vi "S8300E_SetRTCTime_FromPC.vi"() -> ()   [LabVIEW 2011]
panel:
  out "UUT Msg":string
  out "SFCS Msg":string
  out "VISA resource name out":refnum<visa-resource-name>
  out "begin time":u32
  out "toS8300E_RTC_Data":string
  out "PC_Local_Time":string
  out "PC_DATE_STRING":string
  # "設定標準時間\nSetRTC Time from PC  To S8300E"
  # "2015-6-12"
  # "Error Code:RTC\nError Code:UART"
  # "COM9"
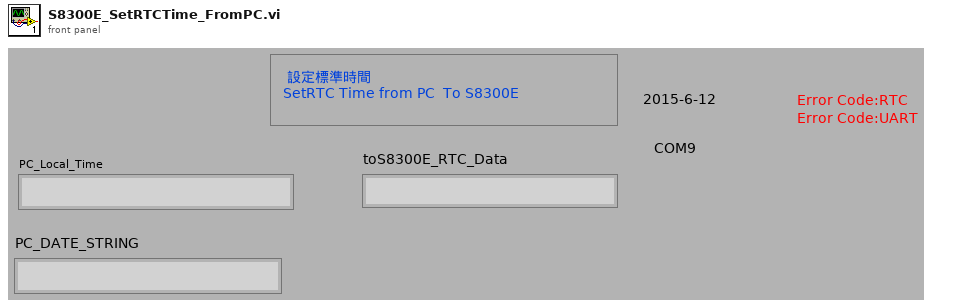
[diagram p1: front panel]
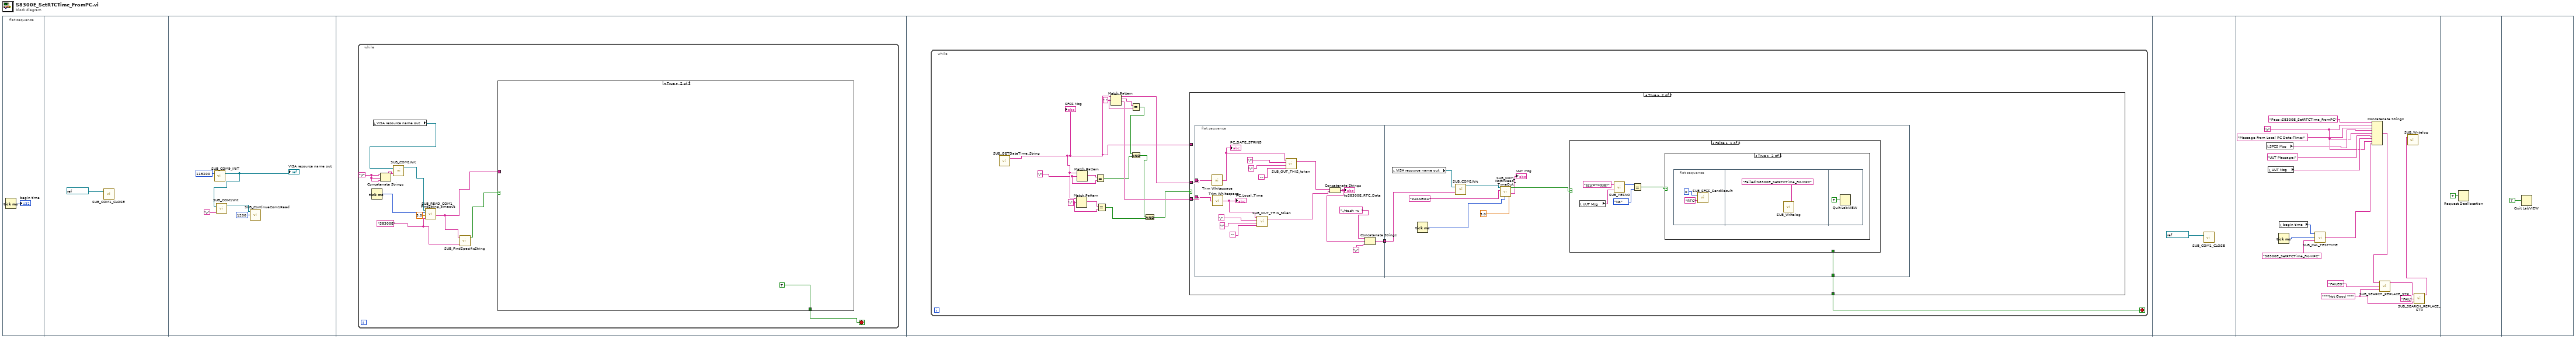
[diagram p0: block diagram]
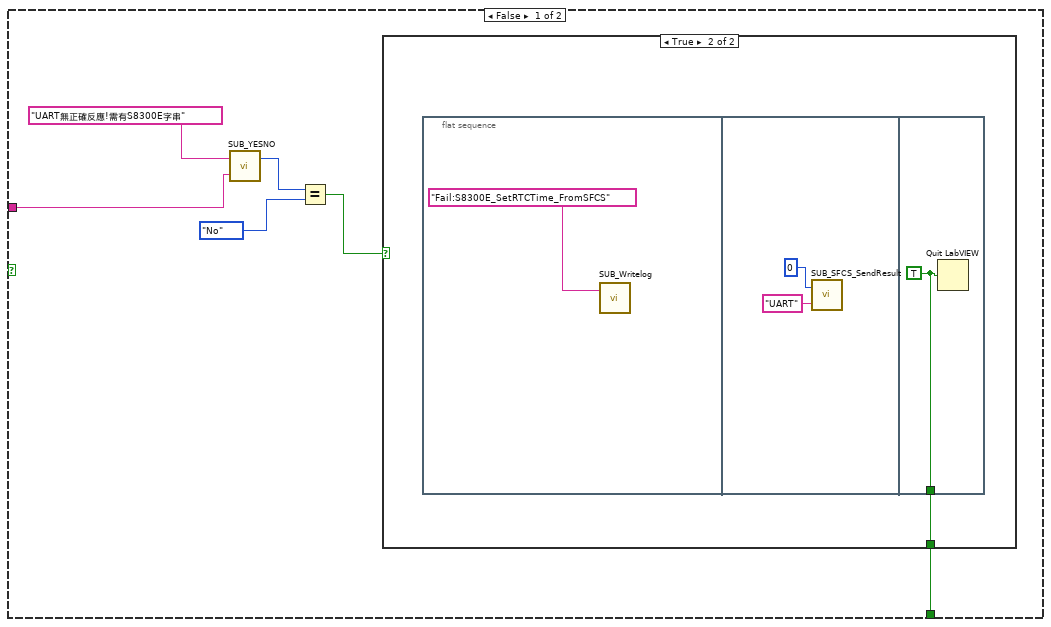
[diagram p2: hidden frame]
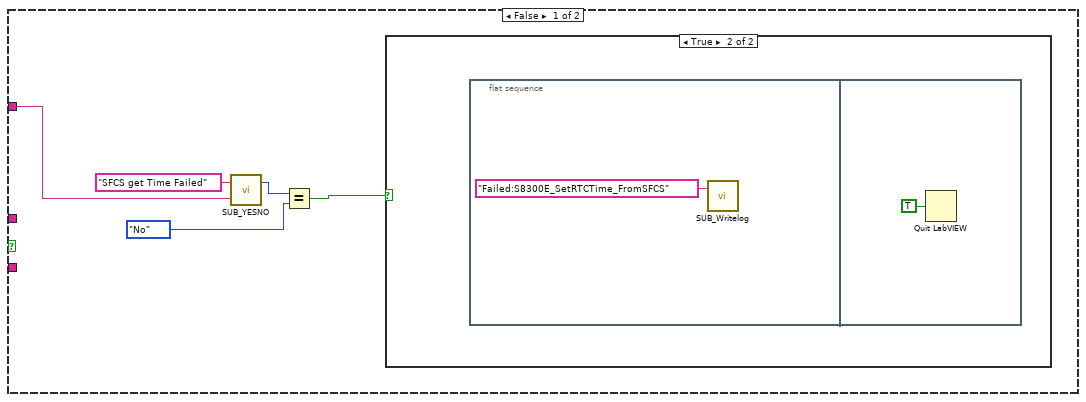
[diagram p4: hidden frame]
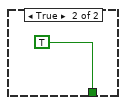
[diagram p7: hidden frame]
diagram:
  n1 = flat-sequence {
    frame #0 {
      n2 = Tick Count (ms)() -> (millisecond timer value=→"begin time":u32)
    }
    frame #1 {
      n3 = call "SUB_COM1_CLOSE.vi"("VISA resource name"=refnum<visa-resource-name> "COM9") -> ()  [unwired: 3 in]
    }
    frame #2 {
      n4 = call "SUB_COM9_INIT.vi"("baud rate"=u32 115200) -> ("VISA resource name out"=w6:refnum<visa-resource-name>)  [unwired: 1 in, 1 out]
      "VISA resource name out" <- w6
      n5 = call "SUB_COM1Wrt.vi"("VISA resource name"=w6, "write buffer"="\r") -> ("duplicate VISA resource name"=w3:refnum<visa-resource-name>)  [unwired: 1 in, 1 out]
      n6 = call "SUB_ContinueCom1Read.vi"("Numeric"=1200, "duplicate VISA resource name 2"=w3) -> ()  [unwired: 1 in, 3 out]
    }
    frame #3 {
      n7 = while {
        stop <- w17 stop-if-true
        w10 = "S8300E" ("Find this String")
        w11 = "\r"
        n8 = Tick Count (ms)() -> (millisecond timer value=w14:u32)
        n9 = local read "VISA resource name out"() -> (w16:refnum<visa-resource-name>)
        n10 = Concatenate Strings(w11, w11, w11) -> (w12:string)
        n11 = call "SUB_COM1Wrt.vi"("VISA resource name"=w16, "write buffer"=w12) -> ("duplicate VISA resource name"=w15:refnum<visa-resource-name>)  [unwired: 1 in, 1 out]
        n12 = call "SUB_READ_COM1_FindString_timeout.vi"("Find this String"=w10, "Timeout Seccond"=3.0, "Begin time"=w14, "duplicate VISA resource name 2"=w15) -> ("Output String"=w9:string)  [unwired: 1 in, 2 out]
        n13 = call "SUB_FindSpecificString.vi"("Find this String"=w10, "String data"=w9) -> ("Found"=w8:bool)  [unwired: 2 in, 1 out]
        n14 = case shown="True" w8 {
          tunnel: w9 -> [w22 _]
          tunnel: [w18 TRUE] -> w17
          frame False {
            n15 = call "SUB_YESNO.vi"("Debug View"=w22, "Status"="UART無正確反應!需有S8300E字串") -> ("yes/no"=w21:enum32{"No Selection", "Yes", "No", "None"})  [unwired: 1 in]
            n16 = Equal?(x=w21, y=enum32{"No Selection", "Yes", "No", "None"}."No") -> (x = y?=w19:bool)
            n17 = case shown="True" w19 {
              tunnel: [_ w24] -> w18
              frame False {
              }
              frame True {
                n18 = flat-sequence {
                  tunnel: [w28] -> w24
                  frame #0 {
                    n19 = call "SUB_Writelog.vi"("Pass/Fail"="Fail:S8300E_SetRTCTime_FromSFCS") -> ()  [unwired: 2 in]
                  }
                  frame #1 {
                    n20 = call "SUB_SFCS_SendResult.vi"("ErrorCode"="UART", "PASS_Fail (1/0)"=i8 0) -> ()  [unwired: 1 out]
                  }
                  frame #2 {
                    w28 = TRUE ("quit? (T)")
                    n21 = Quit LabVIEW(quit? (T)=w28) -> ()
                  }
                }
              }
            }
          }
          frame True {
          }
        }
      }
    }
    frame #4 {
      n22 = while {
        stop <- w33 stop-if-true
        w30 = "/" ("regular expression")
        w38 = ":" ("regular expression")
        w41 = " " ("regular expression")
        n23 = call "SUB_GETDateTime_String.vi"() -> ("date/time string"=w32:string)  [unwired: 3 in]
        "SFCS Msg" <- w32
        n24 = Match Pattern(string=w32, regular expression=w38) -> (match substring=w39:string)  [unwired: 1 in, 3 out]
        n25 = Match Pattern(string=w32, regular expression=w30) -> (match substring=w40:string)  [unwired: 1 in, 3 out]
        n26 = Equal?(x=w40, y=w30) -> (x = y?=w36:bool)
        n27 = Equal?(x=w39, y=w38) -> (x = y?=w31:bool)
        n28 = Match Pattern(string=w32, regular expression=w41) -> (before substring=w44:string, match substring=w42:string, after substring=w43:string)  [unwired: 1 in, 1 out]
        n29 = Equal?(x=w42, y=w41) -> (x = y?=w37:bool)
        n30 = And(x=w37, y=w36) -> (x .and. y?=w35:bool)
        n31 = And(x=w35, y=w31) -> (x .and. y?=w34:bool)
        n32 = case shown="True" w34 {
          tunnel: w44 -> [_ w55]
          tunnel: w43 -> [_ w54]
          tunnel: w32 -> [w45 _]
          tunnel: [_ w53] -> w33
          frame False {
            n33 = call "SUB_YESNO.vi"("Debug View"=w45, "Status"="SFCS get Time Failed") -> ("yes/no"=w48:enum32{"No Selection", "Yes", "No", "None"})  [unwired: 1 in]
            n34 = Equal?(x=w48, y=enum32{"No Selection", "Yes", "No", "None"}."No") -> (x = y?=w46:bool)
            n35 = case shown="True" w46 {
              frame False {
              }
              frame True {
                n36 = flat-sequence {
                  frame #0 {
                    n37 = call "SUB_Writelog.vi"("Pass/Fail"="Failed:S8300E_SetRTCTime_FromSFCS") -> ()  [unwired: 2 in]
                  }
                  frame #1 {
                    n38 = Quit LabVIEW(quit? (T)=TRUE) -> ()
                  }
                }
              }
            }
          }
          frame True {
            n39 = flat-sequence {
              tunnel: w55 -> [w71]
              tunnel: w54 -> [w70]
              tunnel: [w56] -> w52
              tunnel: [w80] -> w53
              tunnel: w52 -> [w78]
              frame #0 {
                n40 = call <vilib>:"Trim Whitespace.vi"("string"=w71) -> ("trimmed string"=w62:string)  [unwired: 1 in]
                "PC_DATE_STRING" <- w62
                n41 = call <vilib>:"Trim Whitespace.vi"("string"=w70) -> ("trimmed string"=w69:string)  [unwired: 1 in]
                "PC_Local_Time" <- w69
                n42 = call "SUB_OUT_THIS_token.vi"("Remove token symbl1 3"="", "Remove token symbl1 2"=":" ("Remove token symbl1"), "Remove token symbl1"="/", "input string"=w69) -> ("result string"=w60:string)  [unwired: 1 in]
                n43 = call "SUB_OUT_THIS_token.vi"("Remove token symbl1 3"="", "Remove token symbl1 2"=":" ("Remove token symbl1"), "Remove token symbl1"="/", "input string"=w62) -> ("result string"=w61:string)  [unwired: 1 in]
                n44 = Concatenate Strings(w61, w60) -> (w57:string)
                "toS8300E_RTC_Data" <- w57
                n45 = Concatenate Strings("./rtc.sh -w  ", w57, "\r") -> (w56:string)
              }
              frame #1 {
                n46 = local read "VISA resource name out"() -> (w79:refnum<visa-resource-name>)
                n47 = Tick Count (ms)() -> (millisecond timer value=w74:u32)
                n48 = call "SUB_COM1Wrt.vi"("VISA resource name"=w79, "write buffer"=w78) -> ("duplicate VISA resource name"=w77:refnum<visa-resource-name>)  [unwired: 1 in, 1 out]
                n49 = call "SUB_COM_NoErrRead_TimeOut.vi"("Timeout Seccond"=5.0, "Begin time"=w74, "Find this String"="PASSED=", "VISA resource name"=w77) -> ("concatenated string"=→"UUT Msg":string, "Found"=w76:bool)  [unwired: 4 in]
                n50 = case shown="False" w76 {
                  tunnel: [_ TRUE] -> w80
                  frame False {
                    n51 = local read "UUT Msg"() -> (w84:string)
                    n52 = call "SUB_YESNO.vi"("Debug View"=w84, "Status"="設定RTC失敗!") -> ("yes/no"=w83:enum32{"No Selection", "Yes", "No", "None"})  [unwired: 1 in]
                    n53 = Equal?(x=w83, y=enum32{"No Selection", "Yes", "No", "None"}."No") -> (x = y?=w81:bool)
                    n54 = case shown="True" w81 {
                      frame False {
                      }
                      frame True {
                        n55 = flat-sequence {
                          frame #0 {
                            n56 = call "SUB_SFCS_SendResult.vi"("ErrorCode"="RTC", "PASS_Fail (1/0)"=i8 0) -> ()  [unwired: 1 out]
                          }
                          frame #1 {
                            n57 = call "SUB_Writelog.vi"("Pass/Fail"="Failed:S8300E_SetRTCTime_FromPC") -> ()  [unwired: 2 in]
                          }
                          frame #2 {
                            n58 = Quit LabVIEW(quit? (T)=TRUE) -> ()
                          }
                        }
                      }
                    }
                  }
                  frame True {
                  }
                }
              }
            }
          }
        }
      }
    }
    frame #5 {
      n59 = call "SUB_COM1_CLOSE.vi"("VISA resource name"=refnum<visa-resource-name> "COM9") -> ()  [unwired: 3 in]
    }
    frame #6 {
      w94 = "***Not Good ***" ("replace string (\"\")")
      w99 = "\r"
      n60 = local read "SFCS Msg"() -> (w102:string)
      n61 = local read "UUT Msg"() -> (w100:string)
      n62 = Tick Count (ms)() -> (millisecond timer value=w106:u32)
      n63 = local read "begin time"() -> (w107:u32)
      n64 = call "SUB_CAL_TESTTIME.vi"("Test Item name"="S8300E_SetRTCTime_FromPC", "Stop tick time"=w106, "Start tick time"=w107) -> ("Test Time output"=w98:string)  [unwired: 2 in]
      n65 = Concatenate Strings("Pass :S8300E_SetRTCTime_FromPC" ("Pass/Fail"), w99, "Message From Local PC Date-Time:", w102, w99, "UUT Message:", w100, w99, w98) -> (w93:string)
      n66 = call "SUB_SEARCH_REPLACE_STR.vi"("replace string (\"\")"=w94, "search string"="FAILED", "input string"=w93) -> ("result string"=w96:string)  [unwired: 2 in]
      n67 = call "SUB_SEARCH_REPLACE_STR.vi"("replace string (\"\")"=w94, "search string"="FAIL", "input string"=w96) -> ("result string"=w92:string)  [unwired: 2 in]
      n68 = call "SUB_Writelog.vi"("Pass/Fail"=w92) -> ()  [unwired: 2 in]
    }
    frame #7 {
      n69 = Request Deallocation(TRUE ("flag")) -> ()
    }
    frame #8 {
      n70 = Quit LabVIEW(quit? (T)=TRUE) -> ()
    }
  }
